vi "Invalid Type.vi"(8 "error in (no error)":errorcluster) -> (0 "error out":errorcluster)   [LabVIEW 2018, in "Application.lvlib" / "Exceptions.lvclass"]
uses:
  Exceptions.lvclass
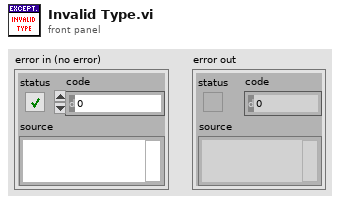
[diagram p1: front panel]
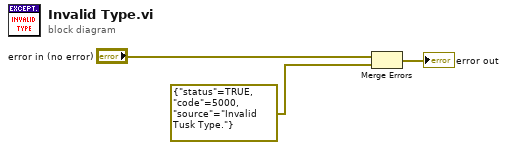
[diagram p0: block diagram]
diagram:
  n1 = Merge Errors("error in (no error)", errorcluster {"status"=TRUE, "code"=5000, "source"="Invalid Tusk Type."} ("error out")) -> (→"error out":errorcluster)
